vi "Dashboard Main.vi"() -> ()   [LabVIEW 2012]
uses:
  <vilib>/event_ctls.llb/eventvkey.ctl
  <vilib>/Utility/config.llb/Read Key (String).vi
  <vilib>/Utility/config.llb/Read Key (I32).vi
  <vilib>/Utility/config.llb/Write Key (String).vi
  <vilib>/Utility/config.llb/Write Key (I32).vi
  <vilib>/Utility/config.llb/NI_LVConfig.lvlib
panel:
  out "Battery Value":dbl(slide) scale=0.0..14.0 scale format="%#_2e"
  out "Battery":sgl(graph)
  in  "Camera Settings":T1={"Frate Rate"=30, "Compression"=30, "Size"=1} {"Frate Rate" scale=1.0..30.0; "Size" items=["640x480", "320x240", "160x120"]}
  out "Mode":T2(ring)=enum."Auto Disabled"
  out "Camera IP":string
  out "JS1 Z":dbl(slide) scale=-1.0..1.0 scale format="%#_2e"
  out "JS2 Z":dbl(slide) scale=-1.0..1.0 scale format="%#_2e"
  out "Joystick 1":cluster{"X":dbl, "Y":dbl}[](graph)
  out "Joystick 2":cluster{"X":dbl, "Y":dbl}[](graph)
  out "JS Buttons 1":T3
  out "JS Buttons 2":T3
  out "MotorSlide4":dbl(slide) scale=-1.0..1.0 scale format="%#_2e"
  out "MotorSlide3":dbl(slide) scale=-1.0..1.0 scale format="%#_2e"
  out "MotorSlide2":dbl(slide) scale=-1.0..1.0 scale format="%#_2e"
  in  "MotorName3":string="Front Left"
  in  "MotorName4":string="Front Right"
  in  "MotorName1":string="Rear Left"
  in  "MotorName2":string="Rear Right"
  out "MotorChart4":dbl(graph)
  out "MotorChart3":dbl(graph)
  out "MotorChart2":dbl(graph)
  out "MotorSlide1":dbl(slide) scale=-1.0..1.0 scale format="%#_2e"
  out "MotorChart1":dbl(graph)
  out "Robot IP":string
  in  "Dashboard Tab":enum32{"Operation", "Test", "Checklist"}(tab)
  out "RectangleZ":dbl
  in  "Angle":dbl
  in  "Checkbox 2":bool
  in  "Checkbox 1":bool
  in  "Slider 1":dbl(slide) scale=0.0..100.0
  in  "Slider":dbl(slide) scale=0.0..100.0 scale format="%#_3g"
  in  "On/Off":bool caption="Solenoid"
  in  "Test Name":u16(ring) items=["Select the test to run...", "Example Test", "-------------------------------", "List of tests is built in robot code.", "Replace with your own automated tests."]
  in  "Test Tree":string(tree)
  in  "Motor":cluster{"Value":dbl, "Enable":bool} {"Value" scale=-1.0..1.0 scale format="%#_3g"}
  out "Progress":T4 {"Test Progress" scale=0.0..100.0}
  in  "Rev/Fwd":cluster{"Forward":bool, "Reverse":bool}
  in  "Ring":u16(ring) items=["Auto", "Fixed indoor", "Fixed outdoor 1", "Fixed outdoor 2", "Fixed fluorescent 1", "Fixed fluorescent 2", "Hold current"]
  in  "Listbox":i32(listbox)
  in  "Viewer":T5(tab)
  out "Mbps":dbl format="%#.1g"
  in  "Enable":bool
  in  "DB Camera Config":bool
  out "Mbps":bool
  out "fps":dbl format="%#.1g"
  out "Image Error Message":string="Timeout in Camera Communications"
  out "Camera Image":T6(plugin-control)
  out "Buttons 1":cluster{"1":bool, "2":bool, "3":bool}
  out "Kinect 1":cluster{"X":dbl, "Y":dbl, "Z":dbl} {"X" scale=1.0..-1.0; "Y" scale=1.0..-1.0; "Z" scale=1.0..-1.0}
  out "Buttons 2":cluster{"1":bool, "2":bool, "3":bool}
  out "Kinect 2":cluster{"X":dbl, "Y":dbl, "Z":dbl} {"X" scale=1.0..-1.0; "Y" scale=1.0..-1.0; "Z" scale=1.0..-1.0}
  out "Version":string
  out "Skeleton Picture":picture
  out "Players":i8
  out "Tree":string(tree)
  # "Drive & Motors"
  # "Robot IP:"
  # "Customize by placing controls and indicators here and name to match\nDashboard Variables on robot."
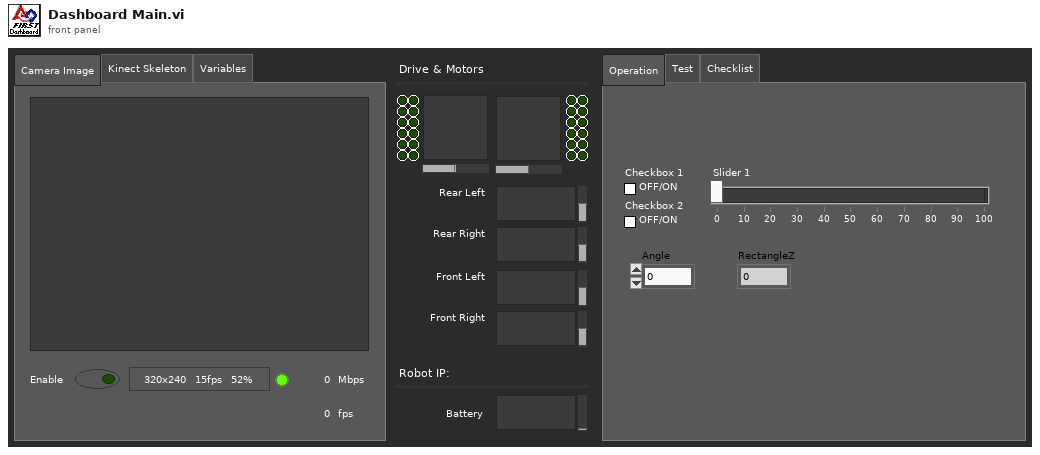
[diagram p1: front panel]
types:
  T1 = cluster{"Frate Rate":i32, "Compression":i32, "Size":u16}
  T2 = enum8{"Tele-Op Disabled", "Tele-Op Enabled", "Auto Disabled", "Auto Enabled", "Test Disabled", "Test Enabled", ""}
  T3 = cluster{bool, bool, bool, bool, bool, bool, bool, bool, bool, bool, bool, bool}
  T4 = cluster{"Test Progress":u8, "Test Progress Text":string}
  T5 = enum32{"Camera Image", "Kinect Skeleton", "Variables"}
  T6 = typedef "IMAQ Image.ctl" = refnum<image>
  T7 = typedef "Image Type" = u32
  T8 = typedef "LVBoundsTypeDef.ctl" = cluster{"Width":u32, "Height":u32}
  T9 = typedef "SkeletonTrackState.ctl" = enum32{"NotTracked", "PositionOnly", "Tracked"}
  T10 = cluster{"TrackingState":u8[], "Position":cluster{"x":sgl, "y":sgl, "z":sgl}, cluster{"x":sgl, "y":sgl, "z":sgl, sgl}[], "TrackState":T9}
  T11 = cluster{cluster{"ScaledToPercentRange":dbl, "ScaledToPercentRange":dbl, "ScaledToPercentRange":dbl}, cluster{bool, bool, bool}}[]
  T12 = cluster{cluster{"ScaledToPercentRange":dbl, "ScaledToPercentRange":dbl, "ScaledToPercentRange":dbl}, cluster{bool, bool, bool}}
  T13 = cluster{"ScaledToPercentRange":dbl, "ScaledToPercentRange":dbl, "ScaledToPercentRange":dbl}
  T14 = typedef "LVRectTypeDef.ctl" = cluster{"Left":i16, "Top":i16, "Right":i16, "Bottom":i16}
  T15 = cluster{"Competition mode":bool, "Robot Link":bool, "Autonomous":bool, "Enabled":bool, "E-Stop":bool, "Simulated":bool, "TestMode":bool, "Docked Window":bool}
  T16 = cluster{"Boolean Array[0]":bool, "Boolean Array[1]":bool, "Boolean Array[2]":bool, "Boolean Array[3]":bool, "Boolean Array[4]":bool, "Boolean Array[5]":bool, "Boolean Array[6]":bool, "Boolean Array[7]":bool, "Boolean Array[8]":bool, "Boolean Array[9]":bool, "Boolean Array[10]":bool, "Boolean Array[11]":bool}
  T17 = typedef "NI_LVConfig.lvlib/Config Data RefNum.ctl" = refnum<k1>
  T18 = typedef "eventvkey.ctl" = enum16{"ASCII", "Enter", "Return", "Shift", "Ctrl", "Alt", "Cmd", "Opt", "Caps", "NumLock", "Clear", "Break", "Up", "Down", "Left", "Right", "Insert", "Delete", "Home", "End", "PageUp", "PageDown", "Escape", "Help", "Pause", "ScrollLock", "F1", "F2", "F3", "F4", "F5", "F6", "F7", "F8", "F9", "F10", "F11", "F12", "F13", "F14", "F15", "F16", "F17", "F18", "F19", "F20", "F21", "F22", "F23", "F24", "Play", "VolumeUp", "VolumeDown", "Mute", "Two Byte Char"}
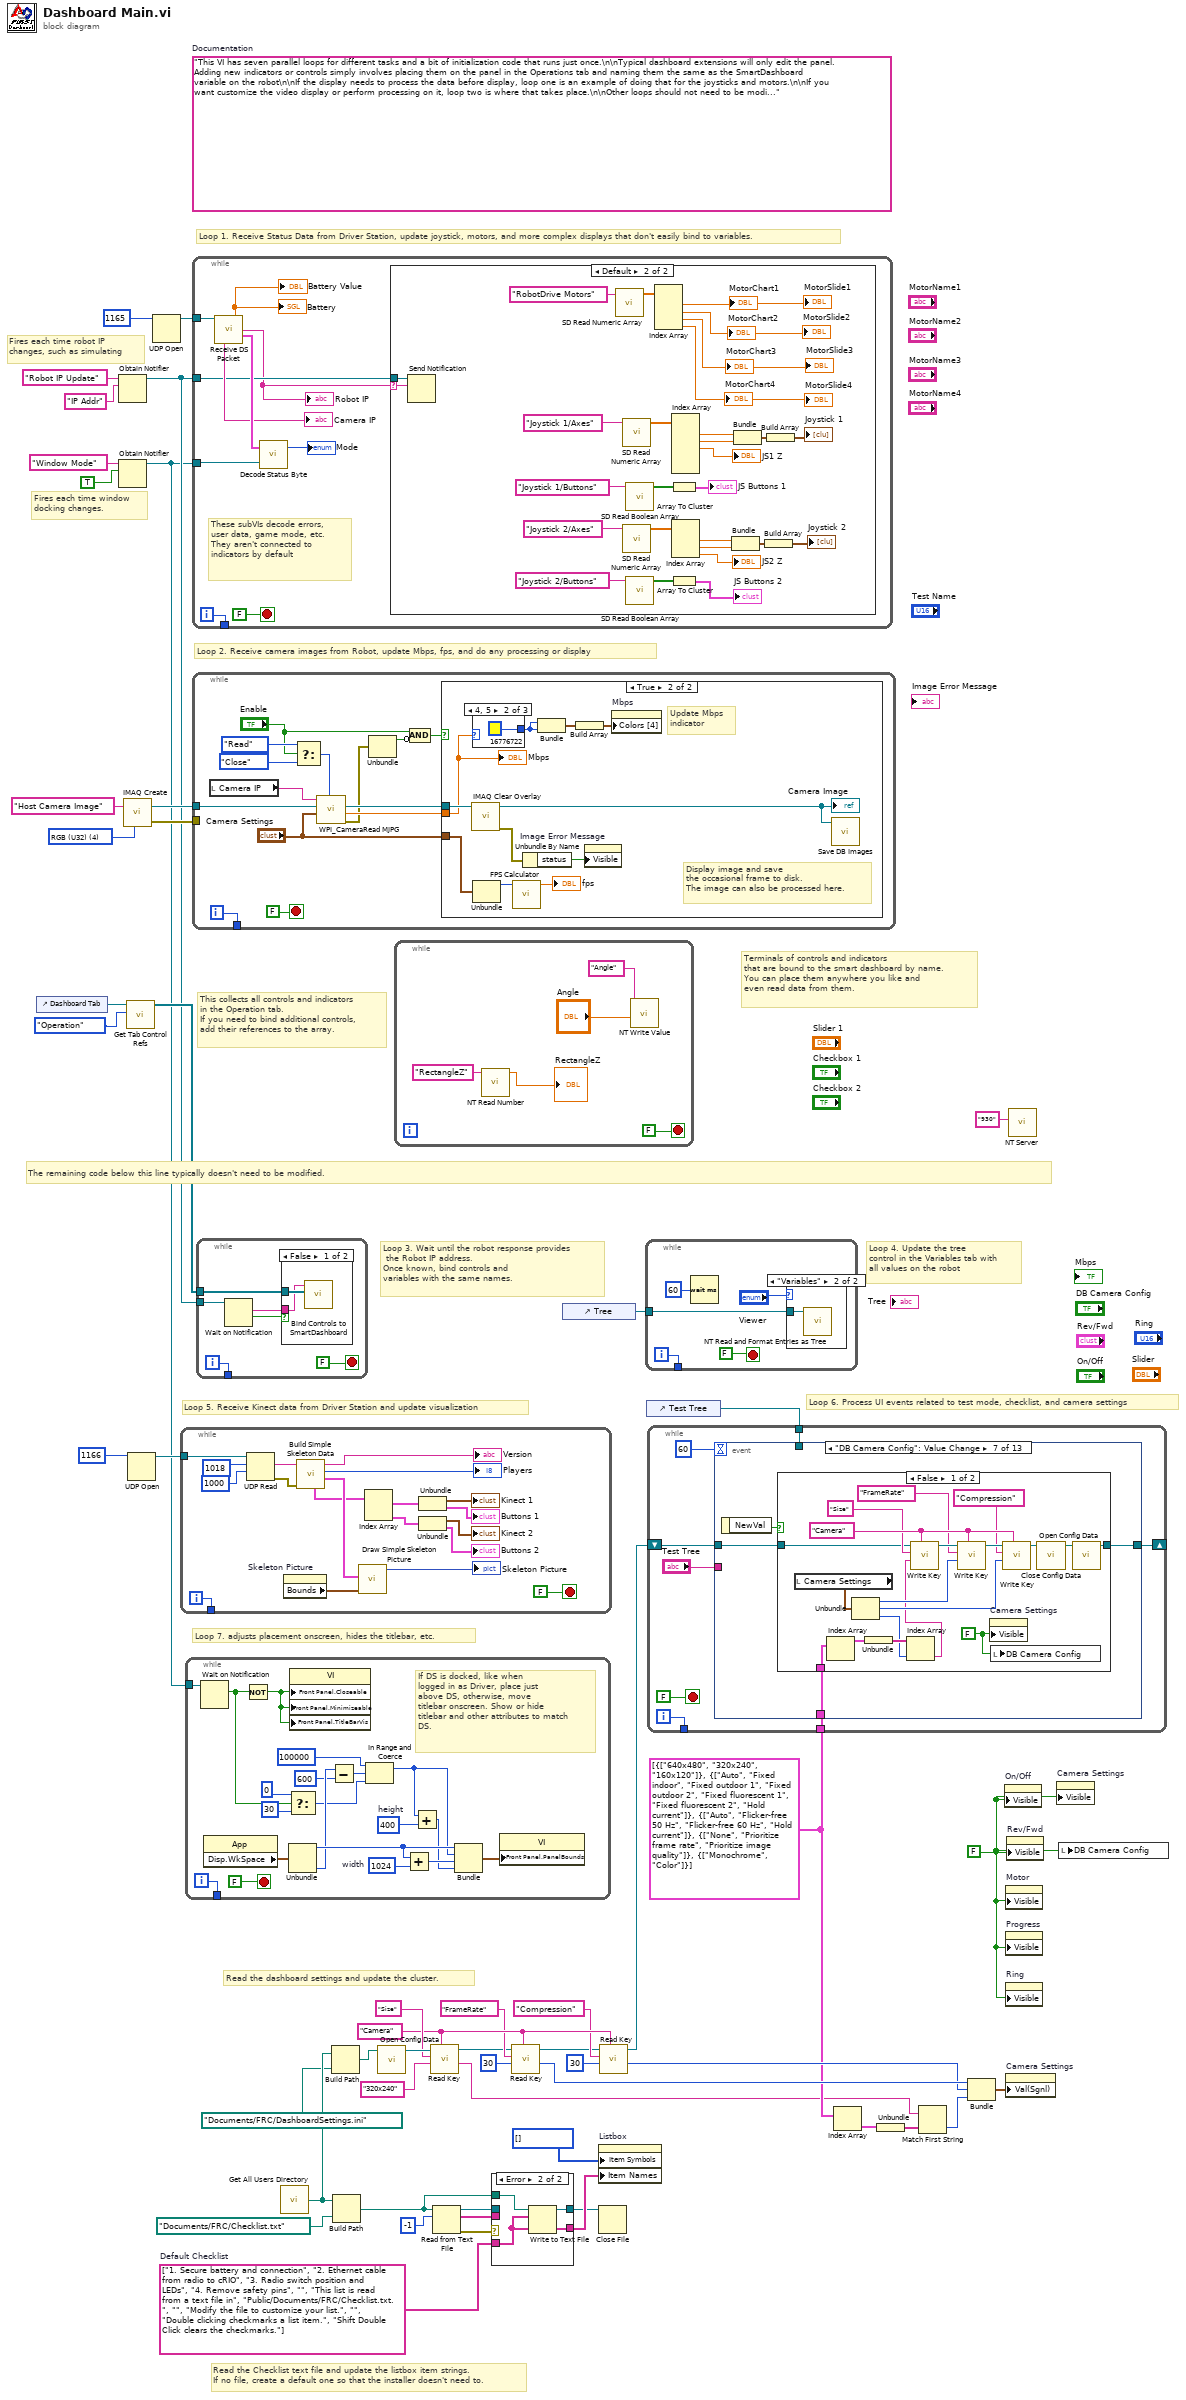
[diagram p0: block diagram]
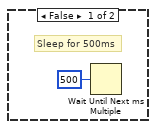
[diagram p3: hidden frame]
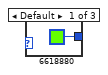
[diagram p4: hidden frame]
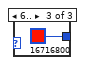
[diagram p5: hidden frame]
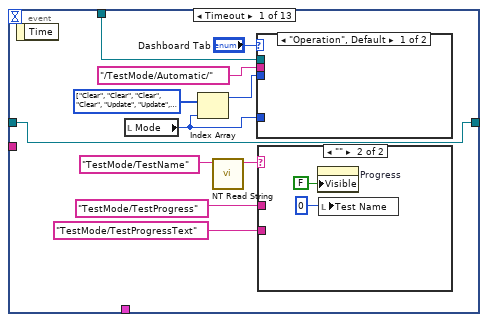
[diagram p7: hidden frame]
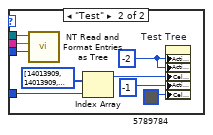
[diagram p8: hidden frame]
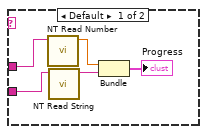
[diagram p9: hidden frame]
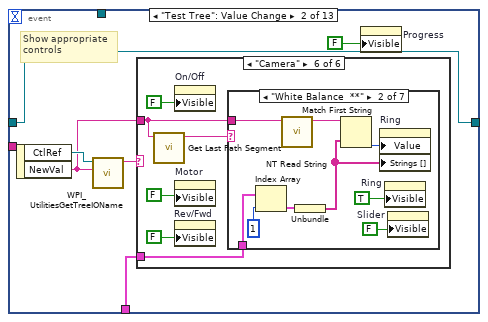
[diagram p10: hidden frame]
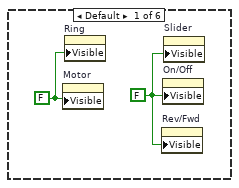
[diagram p11: hidden frame]
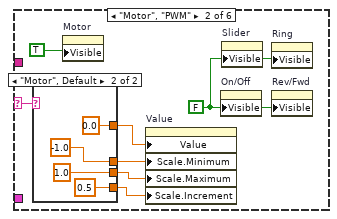
[diagram p12: hidden frame]
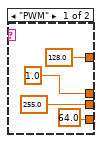
[diagram p13: hidden frame]
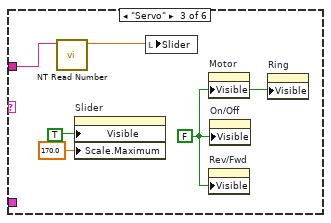
[diagram p14: hidden frame]
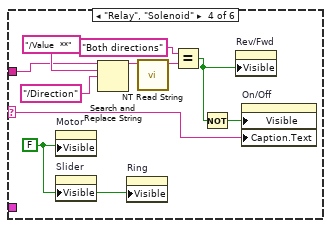
[diagram p15: hidden frame]
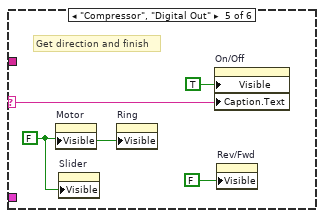
[diagram p16: hidden frame]
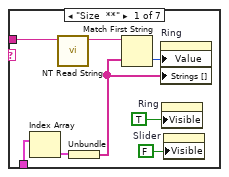
[diagram p17: hidden frame]
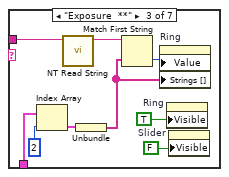
[diagram p18: hidden frame]
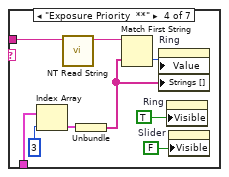
[diagram p19: hidden frame]
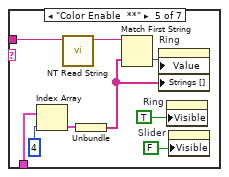
[diagram p20: hidden frame]
diagram:
  w22 = "Camera"
  w14 = cluster{string[]}[] [{["640x480", "320x240", "160x120"]}, {["Auto", "Fixed indoor", "Fixed outdoor 1", "Fixed outdoor 2", "Fixed fluorescent 1", "Fixed fluorescent 2", "Hold current"]}, {["Auto", "Flicker-free 50 Hz", "Flicker-free 60 Hz", "Hold current"]}, {["None", "Prioritize frame rate", "Prioritize image quality"]}, {["Monochrome", "Color"]}]
  w30 = string[] ["1. Secure battery and connection", "2. Ethernet cable from radio to cRIO", "3. Radio switch position and LEDs", "4. Remove safety pins", "", "This list is read from a text file in", "Public/Documents/FRC/Checklist.txt.", "", "Modify the file to customize your list.", "", "Double clicking checkmarks a list item.", "Shift Double Click clears the checkmarks."]  # Default Checklist
  w28 = FALSE ("Visible")
  (unwired) "This VI has seven parallel loops for different tasks and a bit of initialization code that runs just once.\n\nTypical dashboard extensions will only edit the panel. Adding new indicators or controls simply involves placing them on the panel in the Operations tab and naming them the same as the SmartDashboard variable on the robot\n\nIf the display needs to process the data before display, loop one is an example of doing that for the joysticks and motors.\n\nIf you want customize the video display or perform processing on it, loop two is where that takes place.\n\nOther loops should not need to be modified. They are pretty standard, and document the task they perform."  # Documentation
  w51 = T7 4 items=["Grayscale (U8)", "Grayscale (I16)", "Grayscale (SGL)", "Complex (CSG)", "RGB (U32)", "HSL (U32)", "RGB (U64)"] ("Image Type")
  # "Fires each time robot IP\nchanges, such as simulating"
  # "Fires each time window\ndocking changes."
  # "Read the Checklist text file and update the listbox item strings.\nIf no file, create a default one so that the installer doesn't need to."
  # "This collects all controls and indicators\nin the Operation tab.\nIf you need to bind additional controls,\nadd their references to the array."
  # "The remaining code below this line typically doesn't need to be modified."
  # "Loop 6. Process UI events related to test mode, checklist, and camera settings"
  # "Read the dashboard settings and update the cluster."
  # "Terminals of controls and indicators\nthat are bound to the smart dashboard by name.\nYou can place them anywhere you like and\neven read data from them."
  # "Loop 4. Update the tree\ncontrol in the Variables tab with\nall values on the robot"
  # "Loop 3. Wait until the robot response provides\n the Robot IP address.\nOnce known, bind controls and\nvariables with the same names."
  # "Loop 5. Receive Kinect data from Driver Station and update visualization"
  # "Loop 7. adjusts placement onscreen, hides the titlebar, etc."
  # "Loop 1. Receive Status Data from Driver Station, update joystick, motors, and more complex displays that don't easily bind to variables."
  # "Loop 2. Receive camera images from Robot, update Mbps, fps, and do any processing or display"
  n1 = control-ref of="Dashboard Tab"() -> (w44:refnum<vi>)
  n2 = Obtain Notifier(name (unnamed)="Robot IP Update", notification data type="IP Addr" ("name (unnamed)")) -> (notifier out=w41:refnum<notifier>)  [unwired: 2 in, 2 out]
  n3 = Obtain Notifier(name (unnamed)="Window Mode", notification data type=TRUE) -> (notifier out=w34:refnum<notifier>)  [unwired: 2 in, 2 out]
  n4 = call "IMAQ Create"("Image Name"="Host Camera Image", "Image Type"=w51) -> ("New Image"=w49:T6, "error out"=w48:errorcluster)  [unwired: 2 in, 1 out]
  n5 = call <vilib>:"Get Tab Control Refs.vi"("Page Index"=enum32{"Operation", "Test"}."Operation" ("Dashboard Tab"), "TabControl in"=w44) -> ("ControlsOnPage"=w45:refnum<vi>[])  [unwired: 9 in]
  n6 = UDP Open(11:u16 1166 ("port")) -> (port=w46:refnum<k16>)  [unwired: 2 in, 4 out]
  n7 = UDP Open(11:u16 1165 ("port")) -> (port=w52:refnum<k16>)  [unwired: 2 in, 4 out]
  n8 = while {
    tunnel: w46 -> [w70]
    tunnel: [w55] -> _
    i -> [w55]
    stop <- FALSE stop-if-true
    n9 = UDP Read(connection ID=w70, max size (548)=1018 ("bytes to read"), timeout ms (25000)=1000) -> (data out=w64:string, error out=w54:errorcluster)  [unwired: 1 in, 3 out]
    n10 = property on="Skeleton Picture" class="Pict"() -> ("Bounds"=w66:T8)  [unwired: 2 in, 2 out]
    n11 = call "Build Simple Skeleton Data.vi"("error in (no error)"=w54, "data in"=w64) -> ("Skeleton Data"=w65:T10, "NumPlayers"=→"Players":i8, "Version String"=→"Version":string, "Simple Joystick Info"=w62:T11)  [unwired: 5 in, 1 out]
    n12 = call "Draw Simple Skeleton Picture.vi"("Bounds"=w66, "Simple Skeleton"=w65) -> ("new picture out"=→"Skeleton Picture":picture)  [unwired: 9 in]
    n13 = Index Array(array=w62) -> (element #1=w61:T12, element #2=w60:T12)  [unwired: 2 in]
    n14 = Unbundle(w61) -> (→"Kinect 1":T13, →"Buttons 1":cluster{bool, bool, bool})
    n15 = Unbundle(w60) -> (→"Kinect 2":T13, →"Buttons 2":cluster{bool, bool, bool})
  }
  n16 = while {
    tunnel: w34 -> [w91]
    tunnel: [w89] -> _
    i -> [w89]
    stop <- FALSE stop-if-true
    w81 = 1024  # width
    w84 = 400  # height
    # "If DS is docked, like when\nlogged in as Driver, place just\nabove DS, otherwise, move\ntitlebar onscreen. Show or hide\ntitlebar and other attributes to match\nDS."
    n17 = Wait on Notification(notifier=w91) -> (notification=w76:bool)  [unwired: 3 in, 3 out]
    n18 = property class="App"() -> ("Disp.WkSpace"=w87:T14)  [unwired: 2 in, 2 out]
    n19 = Not(x=w76) -> (.not. x?=w90:bool)
    n20 = Unbundle(w87) -> ("Left"=w85:i16, "Bottom"=w82:i16)  [unwired: 2 out]
    n21 = Select(t=0, s=w76, f=30) -> (s? t:f=w75:i32)
    n22 = property class="VI"("Front Panel.Closeable"=w90, "Front Panel.Minimizeable"=w90, "Front Panel.TitleBarVis"=w90) -> ()  [unwired: 2 in, 2 out]
    n23 = Subtract(x=w82, y=600) -> (x-y=w79:i32)
    n24 = In Range and Coerce(upper limit=100000, x=w79, lower limit=w75) -> (coerced(x)=w73:i32)  [unwired: 1 out]
    n25 = Add(x=w85, y=w81) -> (x+y=w86:i32)
    n26 = Add(x=w73, y=w84) -> (x+y=w83:i32)
    n27 = Bundle("Left"=w85, w73, w86, w83) -> (w88:cluster{"Left":i16, i32, i32, i32})  [unwired: 1 out]
    n28 = property class="VI"("Front Panel.PanelBounds"=w88) -> ()  [unwired: 2 in, 2 out]
  }
  n29 = while {
    tunnel: w49 -> [w102]
    tunnel: w48 -> [_]
    tunnel: [w105] -> _
    i -> [w105]
    stop <- FALSE stop-if-true
    n30 = local read "Camera IP"() -> (w104:string)
    n31 = Select(t=enum16{"Read", "Reopen", "Close"}."Read" ("Operation"), s="Enable", f=enum16{"Read", "Reopen", "Close"}."Close" ("Operation")) -> (s? t:f=w97:enum16{"Read", "Reopen", "Close"})
    n32 = call <vilib>:"WPI_CameraRead MJPG.vi"("Operation"=w97, "Camera Settings"="Camera Settings", "Image"=w102, "address"=w104) -> ("error out"=w96:errorcluster, "Bandwidth (kbps)"=w100:dbl, "Image Out"=w101:T6)  [unwired: 5 in]
    n33 = Unbundle(w96) -> ("status"=w94:bool)  [unwired: 2 out]
    n34 = Compound Arithmetic op=AND("Enable", invert w94) -> (w93:bool)
    n35 = case shown="True" w93 {
      tunnel: "Camera Settings" -> [_ w109]
      tunnel: w101 -> [_ w112]
      tunnel: w100 -> [_ w111]
      frame False {
        # "Sleep for 500ms"
        n36 = Wait Until Next ms Multiple(millisecond multiple=u32 500) -> ()  [unwired: 1 out]
      }
      frame True {
        # "Display image and save\nthe occasional frame to disk.\nThe image can also be processed here."
        # "Update Mbps\nindicator"
        n37 = call "IMAQ Clear Overlay"("Image"=w112) -> ("error out"=w117:errorcluster, "Image Out"=w116:T6)  [unwired: 2 in, 7 out]
        "Camera Image" <- w116
        n38 = case shown="4, 5" w111 {
          tunnel: [u32 6618880 ("Color Box") u32 16776722 ("Color Box") u32 16716800 ("Color Box")] -> w113
          frame Default {
          }
          frame 4, 5 {
          }
          frame 6.. {
          }
        }
        n39 = Unbundle(w109) -> ("Frate Rate"=w108:i32)  [unwired: 2 out]
        n40 = call "FPS Calculator.vi"("Average Count"=w108) -> ("fps"=→"fps":dbl)  [unwired: 10 in]
        n41 = Unbundle By Name(w117) -> ("status"=w118:bool)
        n42 = Bundle("Color Box"=w113, "Color Box"=w113) -> (w115:cluster{"Color Box":u32, "Color Box":u32})  [unwired: 1 out]
        n43 = Build Array(w115) -> (w114:cluster{"Color Box":u32, "Color Box":u32}[])
        n44 = property on="Image Error Message" class="Str"("Visible"=w118) -> ()  [unwired: 2 in, 2 out]
        n45 = property on="Mbps" class="Bool (strict)"("Colors [4]"=w114) -> ()  [unwired: 2 in, 2 out]
        n46 = call "Save DB Images.vi"("Image"=w116) -> ()  [unwired: 2 in, 1 out]
        "Mbps" <- w111
      }
    }
  }
  n47 = while {
    tunnel: w52 -> [w129]
    tunnel: w41 -> [w123]
    tunnel: w34 -> [w127]
    tunnel: [w124] -> _
    i -> [w124]
    stop <- FALSE stop-if-true
    # "These subVIs decode errors, user data, game mode, etc.\nThey aren't connected to indicators by default"
    n48 = call "Receive DS Packet.vi"("Recv Socket"=w129) -> ("Battery"=→"Battery" →"Battery Value":sgl, "Robot IP Address"=w122:string, "Status"=w130:T15, "Camera IP Address"=→"Camera IP":string)  [unwired: 1 in, 10 out]
    "Robot IP" <- w122
    n49 = call "Decode Status Byte.vi"("Window Mode Notifier"=w127, "Status"=w130) -> ("Mode"=→"Mode":T2)  [unwired: 1 out]
    n50 = case shown="Default" w122 {
      selector: w122 -> [_ w132]
      tunnel: w123 -> [_ w133]
      frame "0.0.0.0" {
        # "Robot not responding, don't poll the variables"
      }
      frame Default {
        n51 = Send Notification(notification=w132, notifier=w133) -> ()  [unwired: 1 in, 2 out]
        n52 = call <vilib>:"SD Read Numeric Array.vi"("Name"="RobotDrive Motors") -> ("Numeric Array"=w156:dbl[])  [unwired: 8 in, 2 out]
        n53 = call <vilib>:"SD Read Numeric Array.vi"("Name"="Joystick 1/Axes") -> ("Numeric Array"=w149:dbl[])  [unwired: 8 in, 2 out]
        n54 = call <vilib>:"SD Read Numeric Array.vi"("Name"="Joystick 2/Axes") -> ("Numeric Array"=w143:dbl[])  [unwired: 8 in, 2 out]
        n55 = call <vilib>:"SD Read Boolean Array.vi"("Name"="Joystick 1/Buttons") -> ("Boolean Array"=w151:bool[])  [unwired: 8 in, 2 out]
        n56 = call <vilib>:"SD Read Boolean Array.vi"("Name"="Joystick 2/Buttons") -> ("Boolean Array"=w142:bool[])  [unwired: 8 in, 2 out]
        n57 = Index Array(array=w156) -> (element #1=→"MotorChart1" →"MotorSlide1":dbl, element #2=→"MotorSlide2" →"MotorChart2":dbl, element #3=→"MotorChart3" →"MotorSlide3":dbl, element #4=→"MotorChart4" →"MotorSlide4":dbl)  [unwired: 4 in]
        n58 = Array To Cluster(array=w151) -> (cluster=→"JS Buttons 1":T16)
        n59 = Array To Cluster(array=w142) -> (cluster=→"JS Buttons 2":T16)
        n60 = Index Array(array=w149) -> (element #1=w146:dbl, element #2=w147:dbl, element #3=→"JS1 Z":dbl)  [unwired: 6 in, 3 out]
        n61 = Index Array(array=w143) -> (element #1=w138:dbl, element #2=w137:dbl, element #3=→"JS2 Z":dbl)  [unwired: 3 in]
        n62 = Bundle("Numeric"=w138, "Numeric"=w137) -> (w139:cluster{"Numeric":dbl, "Numeric":dbl})  [unwired: 1 in]
        n63 = Bundle("Numeric"=w146, "Numeric"=w147) -> (w145:cluster{"Numeric":dbl, "Numeric":dbl})  [unwired: 1 in]
        n64 = Build Array(w139) -> (→"Joystick 2":cluster{"Numeric":dbl, "Numeric":dbl}[])
        n65 = Build Array(w145) -> (→"Joystick 1":cluster{"Numeric":dbl, "Numeric":dbl}[])
      }
    }
  }
  n66 = while {
    tunnel: w45 -> [w165]
    tunnel: w41 -> [w162]
    tunnel: [w160] -> _
    i -> [w160]
    stop <- FALSE stop-if-true
    n67 = Wait on Notification(notifier=w162) -> (notification=w161:string, timed out?=w163:bool)  [unwired: 3 in, 2 out]
    n68 = case shown="False" w163 {
      tunnel: w165 -> [w167 _]
      tunnel: w161 -> [w166 _]
      frame False {
        n69 = call <vilib>:"Bind Controls to SmartDashboard.vi"("Bound Control Refs"=w167, "Server IP Address"=w166) -> ()  [unwired: 10 in]
      }
      frame True {
      }
    }
  }
  n70 = call "Get All Users Directory.vi"() -> ("All User Path"=w27:path)
  n71 = Build Path(base path=w27, name or relative path=path "Documents/FRC/DashboardSettings.ini") -> (appended path=w26:path)
  n72 = Build Path(base path=w27, name or relative path=path "Documents/FRC/Checklist.txt") -> (appended path=w31:path)
  n73 = call <vilib>:"Open Config Data.vi"("configuration file path"=w26) -> ("refnum"=w25:T17)  [unwired: 8 in, 2 out]
  n74 = while {
    stop <- FALSE stop-if-true
    n75 = call <vilib>:"NT Read Number.vi"("Name"="RectangleZ") -> ("Numeric"=→"RectangleZ":dbl)  [unwired: 9 in, 1 out]
    n76 = call-poly <vilib>:"NT Write Value.vi"("Numeric"="Angle", "Name"="Angle") -> ()  [unwired: 9 in, 1 out]
  }
  n77 = call-poly <vilib>:"Read Key.vi"("section"=w22, "default value"="320x240", "key"="Size", "refnum"=w25) -> ("value"=w12:string, "refnum out"=w7:T17)  [unwired: 2 in, 4 out]
  n78 = Read from Text File(file (use dialog)=w31, count=-1 ("timeout ms (25000)")) -> (refnum out=w9:refnum<file>, text=w32:string[], error out=w33:errorcluster)  [unwired: 2 in, 1 out]
  n79 = case shown="Error" w33 {
    tunnel: w32 -> [w174 _]
    tunnel: [w174 w176] -> w29
    tunnel: w30 -> [_ w176]
    tunnel: w31 -> [_ w177]
    tunnel: [w173 w175] -> w8
    tunnel: w9 -> [w173 _]
    frame No Error {
    }
    frame Error {
      n80 = Write to Text File(file (use dialog)=w177, text=w176) -> (refnum out=w175:refnum<file>)  [unwired: 2 in, 2 out]
    }
  }
  n81 = call-poly <vilib>:"Read Key.vi"("section"=w22, "default value"=30, "key"="FrameRate", "refnum"=w7) -> ("value"=w17:i32, "refnum out"=w6:T17)  [unwired: 1 in, 5 out]
  n82 = control-ref of="Tree"() -> (w3:refnum<vi>)
  n83 = property on="Listbox" class="LstBox (strict)"("Item Symbols"=i32[] [], "Item Names"=w29) -> ()  [unwired: 2 in, 2 out]
  n84 = Close File(refnum=w8) -> ()  [unwired: 1 in, 2 out]
  n85 = call-poly <vilib>:"Read Key.vi"("section"=w22, "default value"=30, "key"="Compression", "refnum"=w6) -> ("value"=w16:i32, "refnum out"=w4:T17)  [unwired: 1 in, 5 out]
  n86 = while {
    tunnel: [w179] -> _
    tunnel: w3 -> [w178]
    i -> [w179]
    stop <- FALSE stop-if-true
    n87 = Wait (ms)(milliseconds to wait=u32 60) -> ()  [unwired: 1 out]
    n88 = case shown="\"Variables\"" "Viewer" {
      tunnel: w178 -> [_ w183]
      frame Default {
      }
      frame "Variables" {
        n89 = call <vilib>:"NT Read and Format Entries as Tree.vi"("Tree Refnum"=w183) -> ()  [unwired: 9 in, 2 out]
      }
    }
  }
  n90 = control-ref of="Test Tree"() -> (w2:refnum<vi>)
  n91 = while {
    tunnel: w14 -> [w188]
    shift-right: [w187] -> _
    shift-left: w4 -> [w186]
    tunnel: [w185] -> _
    tunnel: w2 -> [w184]
    i -> [w185]
    stop <- FALSE stop-if-true
    n92 = event shown="[6] \"DB Camera Config\": Value Change" {
      selector: _ -> [_ _ _ _ _ _ _ _ _ _ _ _ _]
      dyn-events: _ -> [_ _ _ _ _ _ _ _ _ _ _ _ _]
      timeout: u32 60 ("milliseconds to wait") -> [_ _ _ _ _ _ _ _ _ _ _ _ _]
      tunnel: w184 -> [w198 _ _ _ _ _ _ _ _ _ _ _ _]
      tunnel: "Test Tree" -> [_ _ _ _ _ _ _ _ w392 w400 w402 w406 w414]
      tunnel: w188 -> [_ w220 _ _ _ _ w356 w386 _ _ _ _ _]
      tunnel: [w192 w219 _ w322 w330 w342 w355 w379 w391 w398 w401 w405 w413] -> w187
      tunnel: w186 -> [w192 w219 _ w322 w330 w342 w354 w379 w391 w398 w401 w405 w413]
      event Timeout {
        w197 = enum16{"Update", "Clear"}[] [enum."Clear", enum."Clear", enum."Clear", enum."Clear", enum."Update", enum."Update", enum."Clear"] items=["Update", "Clear"]
        n93 = event-data() -> ()  [unwired: 1 in, 1 out]
        n94 = local read "Mode"() -> (w195:T2)
        n95 = Index Array(array=w197, index=w195) -> (element=w196:enum16{"Update", "Clear"})
        n96 = call <vilib>:"NT Read String.vi"("Name"="TestMode/TestName") -> ("String"=w201:string)  [unwired: 9 in, 1 out]
        n97 = case shown="\"Operation\", Default" "Dashboard Tab" {
          tunnel: w198 -> [_ w211]
          tunnel: "/TestMode/Automatic/" ("Name Pattern") -> [_ w210]
          tunnel: w196 -> [_ w209]
          tunnel: w195 -> [_ w207]
          frame "Operation", Default {
          }
          frame "Test" {
            w206 = -2 ("Active Item:Row Number")
            n98 = call <vilib>:"NT Read and Format Entries as Tree.vi"("Operation"=w209, "Name Pattern"=w210, "Tree Refnum"=w211) -> ()  [unwired: 7 in, 2 out]
            n99 = Index Array(array=u32[] [14013909, 14013909, 14013909, 14013909, 14013909, 16777215, 14013909], index=w207) -> (element=w205:u32)
            n100 = property on="Test Tree" class="Tree (strict)"("Active Item Row Number"=w206, "ActiveColNum"=w206, "CellBG"=w205, "Active Item Row Number"=-1 ("Active Item:Row Number"), "CellBG"=u32 5789784 ("Color Box")) -> ()  [unwired: 2 in, 2 out]
          }
        }
        n101 = case shown="\"\"" w201 {
          tunnel: "TestMode/TestProgress" ("Name") -> [w213 _]
          tunnel: "TestMode/TestProgressText" ("Name") -> [w212 _]
          frame Default {
            n102 = call <vilib>:"NT Read Number.vi"("Name"=w213) -> ("Numeric"=w214:dbl)  [unwired: 9 in, 1 out]
            n103 = call <vilib>:"NT Read String.vi"("Name"=w212) -> ("String"=w215:string)  [unwired: 9 in, 1 out]
            n104 = Bundle("Numeric"=w214, "String"=w215) -> (→"Progress":cluster{"Numeric":dbl, "String":string})  [unwired: 1 in]
          }
          frame "" {
            n105 = property on="Progress" class="Clust (strict)"("Visible"=FALSE) -> ()  [unwired: 2 in, 2 out]
            n106 = local write "Test Name"(u16 0) -> ()
          }
        }
      }
      event "Test Tree": Value Change {
        # "Show appropriate\ncontrols"
        n107 = event-data() -> ("CtlRef"=w223:refnum<vi>, "NewVal"=w221:string)  [unwired: 1 in]
        n108 = call <vilib>:"WPI_UtilitiesGetTreeIOName.vi"("NewVal"=w221, "TreeControl in"=w223) -> ("I/O Name"=w224:string)  [unwired: 9 in]
        n109 = case shown="\"Camera\"" w224 {
          selector: w224 -> [_ w231 _ w249 w258 _]
          tunnel: w221 -> [_ _ w246 w248 _ w265]
          tunnel: w220 -> [_ _ _ _ _ w264]
          frame Default {
            w226 = FALSE ("Visible")
            w225 = FALSE ("Visible")
            n110 = property on="Motor" class="Clust (strict)"("Visible"=w225) -> ()  [unwired: 2 in, 2 out]
            n111 = property on="Ring" class="Ring (strict)"("Visible"=w225) -> ()  [unwired: 2 in, 2 out]
            n112 = property on="Rev/Fwd" class="Clust (strict)"("Visible"=w226) -> ()  [unwired: 2 in, 2 out]
            n113 = property on="On/Off" class="Bool (strict)"("Visible"=w226) -> ()  [unwired: 2 in, 2 out]
            n114 = property on="Slider" class="Slide (strict)"("Visible"=w226) -> ()  [unwired: 2 in, 2 out]
          }
          frame "Motor", "PWM" {
            w232 = FALSE ("Visible")
            n115 = case shown="\"Motor\", Default" w231 {
              tunnel: [1.0 ("Value") -1.0 ("Value")] -> w230
              tunnel: [255.0 ("Value") 1.0 ("Value")] -> w229
              tunnel: [128.0 ("Value") 0.0 ("Value")] -> w228
              tunnel: [64.0 ("Value") 0.5 ("Value")] -> w227
              frame "PWM" {
              }
              frame "Motor", Default {
              }
            }
            n116 = property on="Motor" class="Clust (strict)"("Visible"=TRUE) -> ()  [unwired: 2 in, 2 out]
            n117 = property on="Value" class="Slide (strict)"("Value"=w228, "Scale.Minimum"=w230, "Scale.Maximum"=w229, "Scale.Increment"=w227) -> ()  [unwired: 2 in, 2 out]
            n118 = property on="On/Off" class="Bool (strict)"("Visible"=w232) -> ()  [unwired: 2 in, 2 out]
            n119 = property on="Slider" class="Slide (strict)"("Visible"=w232) -> ()  [unwired: 2 in, 2 out]
            n120 = property on="Ring" class="Ring (strict)"("Visible"=w232) -> ()  [unwired: 2 in, 2 out]
            n121 = property on="Rev/Fwd" class="Clust (strict)"("Visible"=w232) -> ()  [unwired: 2 in, 2 out]
          }
          frame "Servo" {
            w244 = FALSE ("Visible")
            n122 = call <vilib>:"NT Read Number.vi"("Name"=w246) -> ("Numeric"=w245:dbl)  [unwired: 9 in, 1 out]
            n123 = property on="Slider" class="Slide (strict)"("Visible"=TRUE, "Scale.Maximum"=170.0 ("Scale.Range:Maximum")) -> ()  [unwired: 2 in, 2 out]
            n124 = local write "Slider"(w245) -> ()
            n125 = property on="Motor" class="Clust (strict)"("Visible"=w244) -> ()  [unwired: 2 in, 2 out]
            n126 = property on="Rev/Fwd" class="Clust (strict)"("Visible"=w244) -> ()  [unwired: 2 in, 2 out]
            n127 = property on="On/Off" class="Bool (strict)"("Visible"=w244) -> ()  [unwired: 2 in, 2 out]
            n128 = property on="Ring" class="Ring (strict)"("Visible"=w244) -> ()  [unwired: 2 in, 2 out]
          }
          frame "Relay", "Solenoid" {
            w247 = FALSE ("Visible")
            n129 = property on="Motor" class="Clust (strict)"("Visible"=w247) -> ()  [unwired: 2 in, 2 out]
            n130 = property on="Slider" class="Slide (strict)"("Visible"=w247) -> ()  [unwired: 2 in, 2 out]
            n131 = Search and Replace String(input string=w248, search string="/Value  **", replace string="/Direction") -> (result string=w254:string)  [unwired: 5 in, 3 out]
            n132 = property on="Ring" class="Ring (strict)"("Visible"=w247) -> ()  [unwired: 2 in, 2 out]
            n133 = call <vilib>:"NT Read String.vi"("Name"=w254) -> ("String"=w252:string)  [unwired: 9 in, 1 out]
            n134 = Equal?(x="Both directions", y=w252) -> (x = y?=w250:bool)
            n135 = Not(x=w250) -> (.not. x?=w251:bool)
            n136 = property on="Rev/Fwd" class="Clust (strict)"("Visible"=w250) -> ()  [unwired: 2 in, 2 out]
            n137 = property on="On/Off" class="Bool (strict)"("Visible"=w251, "Caption.Text"=w249) -> ()  [unwired: 2 in, 2 out]
          }
          frame "Compressor", "Digital Out" {
            w257 = FALSE ("Visible")
            # "Get direction and finish"
            n138 = property on="Motor" class="Clust (strict)"("Visible"=w257) -> ()  [unwired: 2 in, 2 out]
            n139 = property on="Slider" class="Slide (strict)"("Visible"=w257) -> ()  [unwired: 2 in, 2 out]
            n140 = property on="Ring" class="Ring (strict)"("Visible"=w257) -> ()  [unwired: 2 in, 2 out]
            n141 = property on="On/Off" class="Bool (strict)"("Visible"=TRUE, "Caption.Text"=w258) -> ()  [unwired: 2 in, 2 out]
            n142 = property on="Rev/Fwd" class="Clust (strict)"("Visible"=FALSE) -> ()  [unwired: 2 in, 2 out]
          }
          frame "Camera" {
            n143 = call <vilib>:"Get Last Path Segment.vi"("String in"=w265) -> ("String out"=w266:string)  [unwired: 10 in]
            n144 = property on="On/Off" class="Bool (strict)"("Visible"=FALSE) -> ()  [unwired: 2 in, 2 out]
            n145 = property on="Motor" class="Clust (strict)"("Visible"=FALSE) -> ()  [unwired: 2 in, 2 out]
            n146 = property on="Rev/Fwd" class="Clust (strict)"("Visible"=FALSE) -> ()  [unwired: 2 in, 2 out]
            n147 = case shown="\"White Balance  **\"" w266 {
              tunnel: w265 -> [w272 w281 w290 w299 w308 _ w314]
              tunnel: w264 -> [w270 w278 w287 w296 w305 _ _]
              frame "Size  **" {
                n148 = Index Array(array=w270) -> (element=w269:cluster{string[]})  [unwired: 1 in]
                n149 = call <vilib>:"NT Read String.vi"("Name"=w272) -> ("String"=w271:string)  [unwired: 9 in, 1 out]
                n150 = Unbundle(w269) -> (w267:string[])
                n151 = Match First String(2:w267, 3:w271) -> (0:w268:i32)  [unwired: 1 out]
                n152 = property on="Ring" class="Ring (strict)"("Value"=w268, "Strings []"=w267) -> ()  [unwired: 2 in, 2 out]
                n153 = property on="Ring" class="Ring (strict)"("Visible"=TRUE) -> ()  [unwired: 2 in, 2 out]
                n154 = property on="Slider" class="Slide (strict)"("Visible"=FALSE) -> ()  [unwired: 2 in, 2 out]
              }
              frame "White Balance  **" {
                n155 = Index Array(array=w278, index=1) -> (element=w279:cluster{string[]})
                n156 = call <vilib>:"NT Read String.vi"("Name"=w281) -> ("String"=w280:string)  [unwired: 9 in, 1 out]
                n157 = Unbundle(w279) -> (w276:string[])
                n158 = Match First String(2:w276, 3:w280) -> (0:w275:i32)  [unwired: 1 out]
                n159 = property on="Ring" class="Ring (strict)"("Value"=w275, "Strings []"=w276) -> ()  [unwired: 2 in, 2 out]
                n160 = property on="Ring" class="Ring (strict)"("Visible"=TRUE) -> ()  [unwired: 2 in, 2 out]
                n161 = property on="Slider" class="Slide (strict)"("Visible"=FALSE) -> ()  [unwired: 2 in, 2 out]
              }
              frame "Exposure  **" {
                n162 = Index Array(array=w287, index=2) -> (element=w288:cluster{string[]})
                n163 = call <vilib>:"NT Read String.vi"("Name"=w290) -> ("String"=w289:string)  [unwired: 9 in, 1 out]
                n164 = Unbundle(w288) -> (w284:string[])
                n165 = Match First String(2:w284, 3:w289) -> (0:w285:i32)  [unwired: 1 out]
                n166 = property on="Ring" class="Ring (strict)"("Value"=w285, "Strings []"=w284) -> ()  [unwired: 2 in, 2 out]
                n167 = property on="Ring" class="Ring (strict)"("Visible"=TRUE) -> ()  [unwired: 2 in, 2 out]
                n168 = property on="Slider" class="Slide (strict)"("Visible"=FALSE) -> ()  [unwired: 2 in, 2 out]
              }
              frame "Exposure Priority  **" {
                n169 = Index Array(array=w296, index=3) -> (element=w297:cluster{string[]})
                n170 = call <vilib>:"NT Read String.vi"("Name"=w299) -> ("String"=w298:string)  [unwired: 9 in, 1 out]
                n171 = Unbundle(w297) -> (w293:string[])
                n172 = Match First String(2:w293, 3:w298) -> (0:w294:i32)  [unwired: 1 out]
                n173 = property on="Ring" class="Ring (strict)"("Value"=w294, "Strings []"=w293) -> ()  [unwired: 2 in, 2 out]
                n174 = property on="Ring" class="Ring (strict)"("Visible"=TRUE) -> ()  [unwired: 2 in, 2 out]
                n175 = property on="Slider" class="Slide (strict)"("Visible"=FALSE) -> ()  [unwired: 2 in, 2 out]
              }
              frame "Color Enable  **" {
                n176 = Index Array(array=w305, index=4) -> (element=w306:cluster{string[]})
                n177 = call <vilib>:"NT Read String.vi"("Name"=w308) -> ("String"=w307:string)  [unwired: 9 in, 1 out]
                n178 = Unbundle(w306) -> (w302:string[])
                n179 = Match First String(2:w302, 3:w307) -> (0:w303:i32)  [unwired: 1 out]
                n180 = property on="Ring" class="Ring (strict)"("Value"=w303, "Strings []"=w302) -> ()  [unwired: 2 in, 2 out]
                n181 = property on="Ring" class="Ring (strict)"("Visible"=TRUE) -> ()  [unwired: 2 in, 2 out]
                n182 = property on="Slider" class="Slide (strict)"("Visible"=FALSE) -> ()  [unwired: 2 in, 2 out]
              }
              frame Default {
                n183 = property on="Ring" class="Ring (strict)"("Visible"=FALSE) -> ()  [unwired: 2 in, 2 out]
                n184 = property on="Slider" class="Slide (strict)"("Visible"=FALSE) -> ()  [unwired: 2 in, 2 out]
              }
              frame "Brightness  **", "Color Level  **", "Compression  **", "FPS  **", "Sharpness  **" {
                n185 = call <vilib>:"NT Read Number.vi"("Name"=w314) -> ("Numeric"=w313:dbl)  [unwired: 9 in, 1 out]
                n186 = local write "Slider"(w313) -> ()
                n187 = property on="Slider" class="Slide (strict)"("Visible"=TRUE, "Scale.Maximum"=100.0 ("Scale.Range:Maximum")) -> ()  [unwired: 2 in, 2 out]
                n188 = property on="Ring" class="Ring (strict)"("Visible"=FALSE) -> ()  [unwired: 2 in, 2 out]
              }
            }
          }
        }
        n189 = property on="Progress" class="Clust (strict)"("Visible"=FALSE) -> ()  [unwired: 2 in, 2 out]
      }
      event "Test Name": Mouse Enter {
        # "Populate the ring with the list of tests"
        n190 = event-data() -> ()  [unwired: 1 in, 1 out]
        n191 = call <vilib>:"NT Read String Array.vi"("Name"="TestMode/TestList") -> ("String Array"=w321:string[])  [unwired: 9 in, 1 out]
        n192 = Build Array (concatenate)("Select the test to run...", w321) -> (w320:string[])
        n193 = property on="Test Name" class="Ring (strict)"("Strings []"=w320) -> ()  [unwired: 2 in, 2 out]
      }
      event "Test Name": Value Change {
        w323 = FALSE ("Visible")
        # "Tell the robot the test name to run"
        n194 = event-data() -> ("NewVal"=w327:u16)  [unwired: 1 in]
        n195 = property on="Test Name" class="Ring (strict)"() -> ("Strings []"=w328:string[])  [unwired: 2 in, 2 out]
        n196 = local write "Progress"(T4 {"Test Progress"=0, "Test Progress Text"=""} ("Progress")) -> ()
        n197 = Index Array(array=w328, index=w327) -> (element=w326:string)
        n198 = call <vilib>:"NT Write String.vi"("String"=w326, "Name"="TestMode/TestName") -> ()  [unwired: 9 in, 1 out]
        n199 = property on="Progress" class="Clust (strict)"("Visible"=TRUE) -> ()  [unwired: 2 in, 2 out]
        n200 = property on="Motor" class="Clust (strict)"("Visible"=w323) -> ()  [unwired: 2 in, 2 out]
        n201 = property on="Slider" class="Slide (strict)"("Visible"=w323) -> ()  [unwired: 2 in, 2 out]
        n202 = property on="On/Off" class="Bool (strict)"("Visible"=w323) -> ()  [unwired: 2 in, 2 out]
        n203 = property on="Rev/Fwd" class="Clust (strict)"("Visible"=w323) -> ()  [unwired: 2 in, 2 out]
        n204 = property on="Ring" class="Ring (strict)"("Visible"=w323) -> ()  [unwired: 2 in, 2 out]
      }
      event "Listbox": Double Click {
        n205 = event-data() -> ("PlatMods.Shift"=w331:bool, "Row"=w333:i32)  [unwired: 1 in]
        n206 = case shown="False" w331 {
          tunnel: w333 -> [w337 _]
          tunnel: 1 -> [w336 _]
          frame False {
            n207 = property on="Listbox" class="LstBox (strict)"() -> ("Item Symbols"=w335:i32[])  [unwired: 2 in, 2 out]
            n208 = Replace Array Subset(array=w335, new element=w336, index=w337) -> (w334:i32[])
            n209 = property on="Listbox" class="LstBox (strict)"("Item Symbols"=w334) -> ()  [unwired: 2 in, 2 out]
          }
          frame True {
            w338 = 0 ("Top Row")
            n210 = property on="Listbox" class="LstBox (strict)"() -> ("Number of Rows"=w340:u32)  [unwired: 2 in, 2 out]
            n211 = Initialize Array(0, w340) -> (w339:i32[])
            n212 = property on="Listbox" class="LstBox (strict)"("Top Row"=w338, "Value"=w338, "Item Symbols"=w339) -> ()  [unwired: 2 in, 2 out]
          }
        }
      }
      event "Listbox": Key Down {
        n213 = event-data() -> ("VKey"=w344:T18)  [unwired: 1 in]
        n214 = case shown="\"Left\", \"Right\"" w344 {
          selector: w344 -> [w349 _]
          tunnel: eventvkey."Left" ("VKey") -> [w347 _]
          frame "Left", "Right" {
            n215 = Equal?(x=w347, y=w349) -> (x = y?=w348:bool)
            n216 = Select(t=0, s=w348, f=1) -> (s? t:f=w350:i32)
            n217 = property on="Listbox" class="LstBox (strict)"() -> ("Item Symbols"=w353:i32[])  [unwired: 2 in, 2 out]
            n218 = Replace Array Subset(array=w353, new element=w350, index="Listbox") -> (w352:i32[])
            n219 = property on="Listbox" class="LstBox (strict)"("Item Symbols"=w352) -> ()  [unwired: 2 in, 2 out]
          }
          frame Default {
          }
        }
      }
      event "DB Camera Config": Value Change {
        n220 = event-data() -> ("NewVal"=w357:bool)  [unwired: 1 in]
        n221 = case shown="False" w357 {
          tunnel: w356 -> [w366 _]
          tunnel: [w359 w377] -> w355
          tunnel: w354 -> [w358 w377]
          frame False {
            w373 = "Camera"
            w376 = FALSE ("Visible")
            n222 = local read "Camera Settings"() -> (w365:T1)
            n223 = Index Array(array=w366) -> (element=w369:cluster{string[]})  [unwired: 1 in]
            n224 = Unbundle(w365) -> ("Frate Rate"=w364:i32, "Compression"=w363:i32, "Size"=w367:u16)
            n225 = Unbundle(w369) -> (w368:string[])
            n226 = Index Array(array=w368, index=w367) -> (element=w362:string)
            n227 = call-poly <vilib>:"Write Key.vi"("section"=w373, "value"=w362, "key"="Size", "refnum"=w358) -> ("refnum out"=w375:T17)  [unwired: 2 in, 5 out]
            n228 = call-poly <vilib>:"Write Key.vi"("section"=w373, "value"=w364, "key"="FrameRate", "refnum"=w375) -> ("refnum out"=w374:T17)  [unwired: 1 in, 6 out]
            n229 = property on="Camera Settings" class="Clust (strict)"("Visible"=w376) -> ()  [unwired: 2 in, 2 out]
            n230 = local write "DB Camera Config"(w376) -> ()
            n231 = call-poly <vilib>:"Write Key.vi"("section"=w373, "value"=w363, "key"="Compression", "refnum"=w374) -> ("refnum out"=w360:T17)  [unwired: 1 in, 6 out]
            n232 = call <vilib>:"Close Config Data.vi"("refnum"=w360) -> ("file path"=w361:path)  [unwired: 2 in, 8 out]
            n233 = call <vilib>:"Open Config Data.vi"("configuration file path"=w361) -> ("refnum"=w359:T17)  [unwired: 8 in, 2 out]
          }
          frame True {
            n234 = property on="Camera Settings" class="Clust (strict)"("Visible"=TRUE) -> ()  [unwired: 2 in, 2 out]
          }
        }
      }
      event "Camera Settings": Value Change {
        n235 = event-data() -> ("NewVal"=w390:T1)  [unwired: 1 in]
        n236 = Index Array(array=w386) -> (element=w385:cluster{string[]})  [unwired: 1 in]
        n237 = Unbundle(w390) -> ("Frate Rate"=w381:i32, "Compression"=w380:i32, "Size"=w383:u16)
        n238 = Unbundle(w385) -> (w384:string[])
        n239 = Index Array(array=w384, index=w383) -> (element=w382:string)
        n240 = Format Into String(format string="%s   %dfps   %d%%", w382, w381, w380) -> (resulting string=w387:string)  [unwired: 2 in, 1 out]
        n241 = Build Array(w387) -> (w388:string[])
        n242 = property on="DB Camera Config" class="Bool (strict)"("Strings [4]"=w388) -> ()  [unwired: 2 in, 2 out]
      }
      event "Motor.Enable": Value Change {
        n243 = event-data() -> ("NewVal"=w396:bool)  [unwired: 1 in]
        n244 = Unbundle("Motor") -> ("Value"=w395:dbl)  [unwired: 1 out]
        n245 = Select(t=w395, s=w396, f=0.0) -> (s? t:f=w393:dbl)
        n246 = call <vilib>:"NT Write Number.vi"("Numeric"=w393, "Name"=w392) -> ()  [unwired: 9 in, 1 out]
      }
      event "Slider": Value Change {
        n247 = event-data() -> ("NewVal"=w399:dbl)  [unwired: 1 in]
        n248 = call <vilib>:"NT Write Number.vi"("Numeric"=w399, "Name"=w400) -> ()  [unwired: 9 in, 1 out]
      }
      event "On/Off": Value Change {
        n249 = event-data() -> ("NewVal"=w404:bool)  [unwired: 1 in]
        n250 = Boolean To (0,1)(Boolean=w404) -> (0, 1=w403:i16)
        n251 = call <vilib>:"NT Write Number.vi"("Numeric"=w403, "Name"=w402) -> ()  [unwired: 9 in, 1 out]
      }
      event "Rev/Fwd": Value Change {
        n252 = event-data() -> ("NewVal.Forward"=w412:bool, "NewVal.Reverse"=w411:bool)  [unwired: 1 in]
        n253 = Boolean To (0,1)(Boolean=w412) -> (0, 1=w408:i16)
        n254 = Boolean To (0,1)(Boolean=w411) -> (0, 1=w410:i16)
        n255 = Negate(x=w410) -> (-x=w409:i16)
        n256 = Add(x=w408, y=w409) -> (x+y=w407:i16)
        n257 = call <vilib>:"NT Write Number.vi"("Numeric"=w407, "Name"=w406) -> ()  [unwired: 9 in, 1 out]
      }
      event "Ring": Value Change {
        n258 = event-data() -> ("NewVal"=w416:u16)  [unwired: 1 in]
        n259 = property on="Ring" class="Ring (strict)"() -> ("Strings []"=w417:string[])  [unwired: 2 in, 2 out]
        n260 = Index Array(array=w417, index=w416) -> (element=w415:string)
        n261 = call <vilib>:"NT Write String.vi"("String"=w415, "Name"=w414) -> ()  [unwired: 9 in, 1 out]
      }
    }
  }
  n262 = Index Array(array=w14) -> (element=w15:cluster{string[]})  [unwired: 1 in]
  n263 = Unbundle(w15) -> (w13:string[])
  n264 = Match First String(2:w13, 3:w12) -> (0:w11:i32)  [unwired: 1 out]
  n265 = Bundle("value"=w17, "value"=w16, "index"=w11) -> (w5:cluster{"value":i32, "value":i32, "index":i32})  [unwired: 1 out]
  n266 = property on="On/Off" class="Bool (strict)"("Visible"=w28) -> ()  [unwired: 2 in, 2 out]
  n267 = property on="Motor" class="Clust (strict)"("Visible"=w28) -> ()  [unwired: 2 in, 2 out]
  n268 = property on="Progress" class="Clust (strict)"("Visible"=w28) -> ()  [unwired: 2 in, 2 out]
  n269 = property on="Ring" class="Ring (strict)"("Visible"=w28) -> ()  [unwired: 2 in, 2 out]
  n270 = property on="Camera Settings" class="Clust (strict)"("Val(Sgnl)"=w5) -> ()  [unwired: 2 in, 2 out]
  n271 = property on="Rev/Fwd" class="Clust (strict)"("Visible"=w28) -> ()  [unwired: 2 in, 2 out]
  n272 = call <vilib>:"NT Server.vi"("Server Name"="930") -> ()  [unwired: 11 in]
  n273 = property on="Camera Settings" class="Clust (strict)"("Visible"=w28) -> ()  [unwired: 2 in, 2 out]
  n274 = local write "DB Camera Config"(w28) -> ()
